vi "Enable Output.vi"(5 "Channel (3:3)":u16(ring)=1 items=["1"=1, "2"=2, "3"=3], 6 "Channel (2:2)":u16(ring)=1 items=["1"=1, "2"=2, "3"=3], 8 "error in (no error)":errorcluster, 9 "Enable Output (F: False)":bool, 10 "Channel (1:1)":u16(ring)=1 items=["1"=1, "2"=2, "3"=3], 11 "VISA resource name":refnum<visa-resource-name>) -> (0 "error out":errorcluster, 3 "VISA resource name out":refnum<visa-resource-name>)   [LabVIEW 2017, in "BK Precision 913XX.lvlib"]
doc: "Enables or Disables the output of one selectable channel or all channels."
uses:
  <instrlib>/BK Precision 913XX/BK Precision 913XX.lvlib
panel:
  in  "Control Mode (0:Single)":u16(ring) items=["Single", "All"]
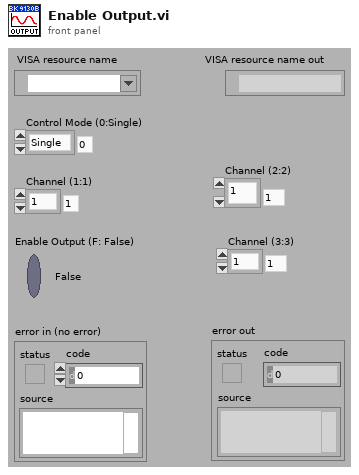
[diagram p1: front panel]
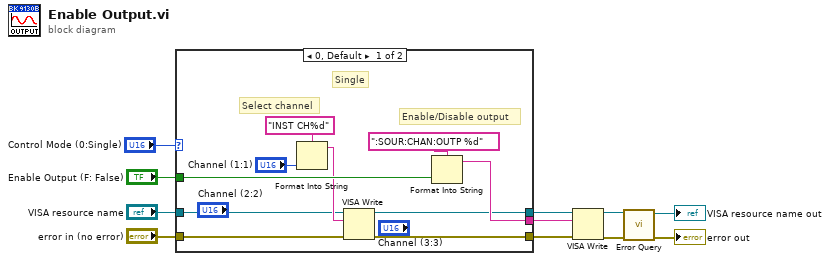
[diagram p0: block diagram]
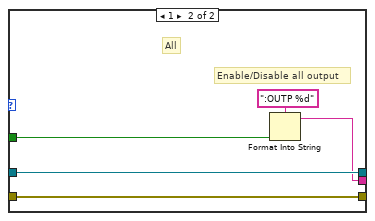
[diagram p2: hidden frame]
diagram:
  n1 = case shown="0, Default" "Control Mode (0:Single)" {
    tunnel: "Enable Output (F: False)" -> [w20 w24]
    tunnel: [w19 w22] -> w8
    tunnel: "VISA resource name" -> [w16 w26]
    tunnel: "error in (no error)" -> [w15 w25]
    tunnel: [w14 w25] -> w3
    tunnel: [w13 w26] -> w2
    frame 0, Default {
      # "Single"
      # "Select channel"
      # "Enable/Disable output"
      n2 = Format Into String(format string="INST CH%d", "Channel (1:1)") -> (resulting string=w17:string)  [unwired: 2 in, 1 out]
      n3 = VISA Write(VISA resource name=w16, write buffer=w17, error in (no error)=w15) -> (VISA resource name out=w13:refnum<visa-resource-name>, error out=w14:errorcluster)  [unwired: 1 out]
      n4 = Format Into String(format string=":SOUR:CHAN:OUTP %d", w20) -> (resulting string=w19:string)  [unwired: 2 in, 1 out]
    }
    frame 1 {
      # "Enable/Disable all output"
      # "All"
      n5 = Format Into String(format string=":OUTP %d", w24) -> (resulting string=w22:string)  [unwired: 2 in, 1 out]
    }
  }
  n6 = VISA Write(VISA resource name=w2, write buffer=w8, error in (no error)=w3) -> (VISA resource name out=w7:refnum<visa-resource-name>, error out=w6:errorcluster)  [unwired: 1 out]
  n7 = call <instrlib>:"Error Query.vi"("error in (no error)"=w6, "VISA resource name"=w7) -> ("error out"=→"error out":errorcluster, "VISA resource name out"=→"VISA resource name out":refnum<visa-resource-name>)  [unwired: 6 in, 2 out]
